vi "PIC3_DEMO.vi"() -> ()   [LabVIEW 2016]
panel:
  in  "subset rect":T1
  out "new picture 2":picture
  out "new picture":picture
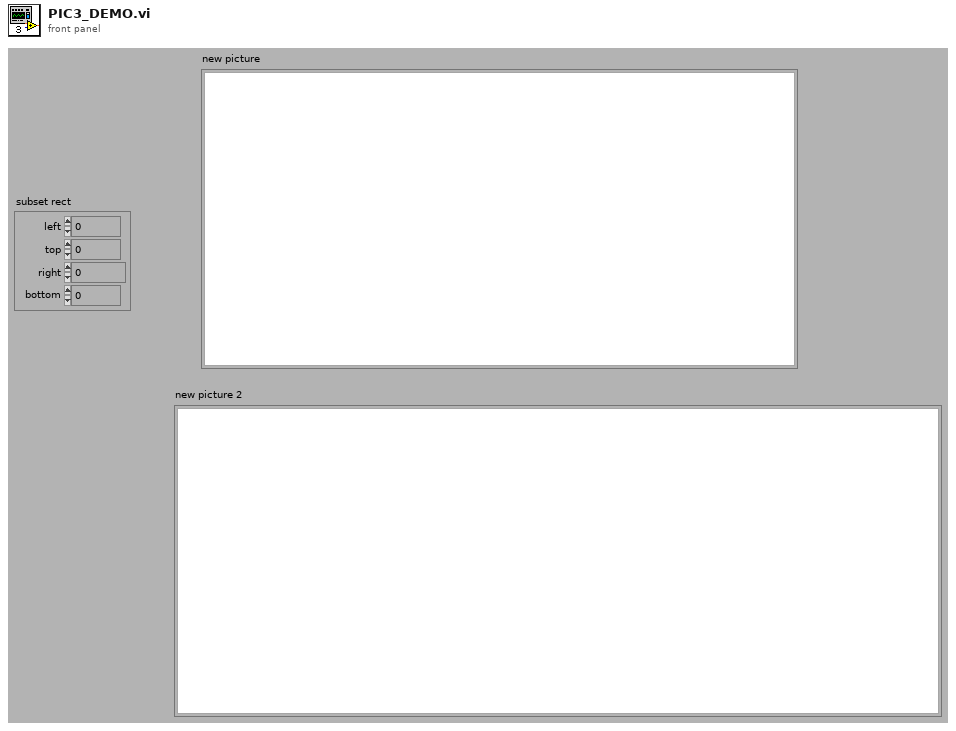
[diagram p1: front panel]
types:
  T1 = cluster{"left":i16, "top":i16, "right":i16, "bottom":i16}
  T2 = typedef "imagedata.ctl" = cluster{"image type":i32, "image depth":i32, "image":u8[], "mask":u8[], "colors":u32[], "Rectangle":cluster{"left":i16, "top":i16, "right":i16, "bottom":i16}}
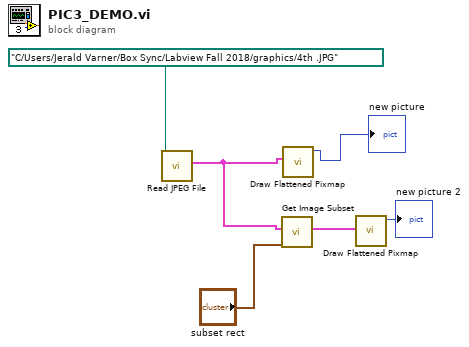
[diagram p0: block diagram]
diagram:
  n1 = call <vilib>:"Read JPEG File.vi"("path to JPEG file"=path "C:/Users/Jerald Varner/Box Sync/Labview Fall 2018/graphics/4th .JPG" ("path to JPEG file 2")) -> ("image data"=w6:T2)  [unwired: 8 in, 2 out]
  n2 = call <vilib>:"Get Image Subset.vi"("subset rect"="subset rect", "image data"=w6) -> ("image subset"=w5:T2)  [unwired: 4 in, 1 out]
  n3 = call <vilib>:"Draw Flattened Pixmap.vi"("image data"=w6) -> ("new picture"=→"new picture":picture)  [unwired: 8 in]
  n4 = call <vilib>:"Draw Flattened Pixmap.vi"("image data"=w5) -> ("new picture"=→"new picture 2":picture)  [unwired: 8 in]
